vi "thermal_optical_camera_2.vi"() -> ()   [LabVIEW 2025]
panel:
  out "file name out":string
  in  "File Path":string="C:\\Digambar\\Metal_thin_wall\\Optical_images\\Optical_images"
  in  "Stop (F)":bool
  in  "Acquisition Control:\nExposure Time [100, 3E7]":dbl=999.0 caption="Acquisition Control::Exposure Time" min=100.0 max=29999995.0
  in  "Analog Control:\nGain [0, 27]":dbl caption="Analog Control::Gain" min=0.0 max=27.045663671679687
  in  "Analog Control:\nBlack Level [-5, 10]":dbl caption="Analog Control::Black Level" min=-5.0000011920928955 max=10.000002384185791
  in  "Analog Control:\nGamma [0.25, 4.00]":dbl=0.800048828125 caption="Analog Control::Gamma" min=0.25 max=4.0 step=0.05
  out "Optical camera":T1(plugin-control)
  in  "optical capture interval (s)":dbl
  in  "thermal capture interval (s)":dbl
  out "Thermal camera":T1(plugin-control)
  out "IP address":string
  out "Output":string
  in  "Flag Button":bool
  in  "Stop Recording":bool
  in  "Stop Preview":bool
  in  "Focus":dbl(slide) scale=0.0..100.0
  in  "Record":bool
  # "Destination for Optical Images:"
  # "change folder names each time you run,\nso it saves data sets in dedicated folders:\nfolder1\nfolder2\nfolder3\netc..."
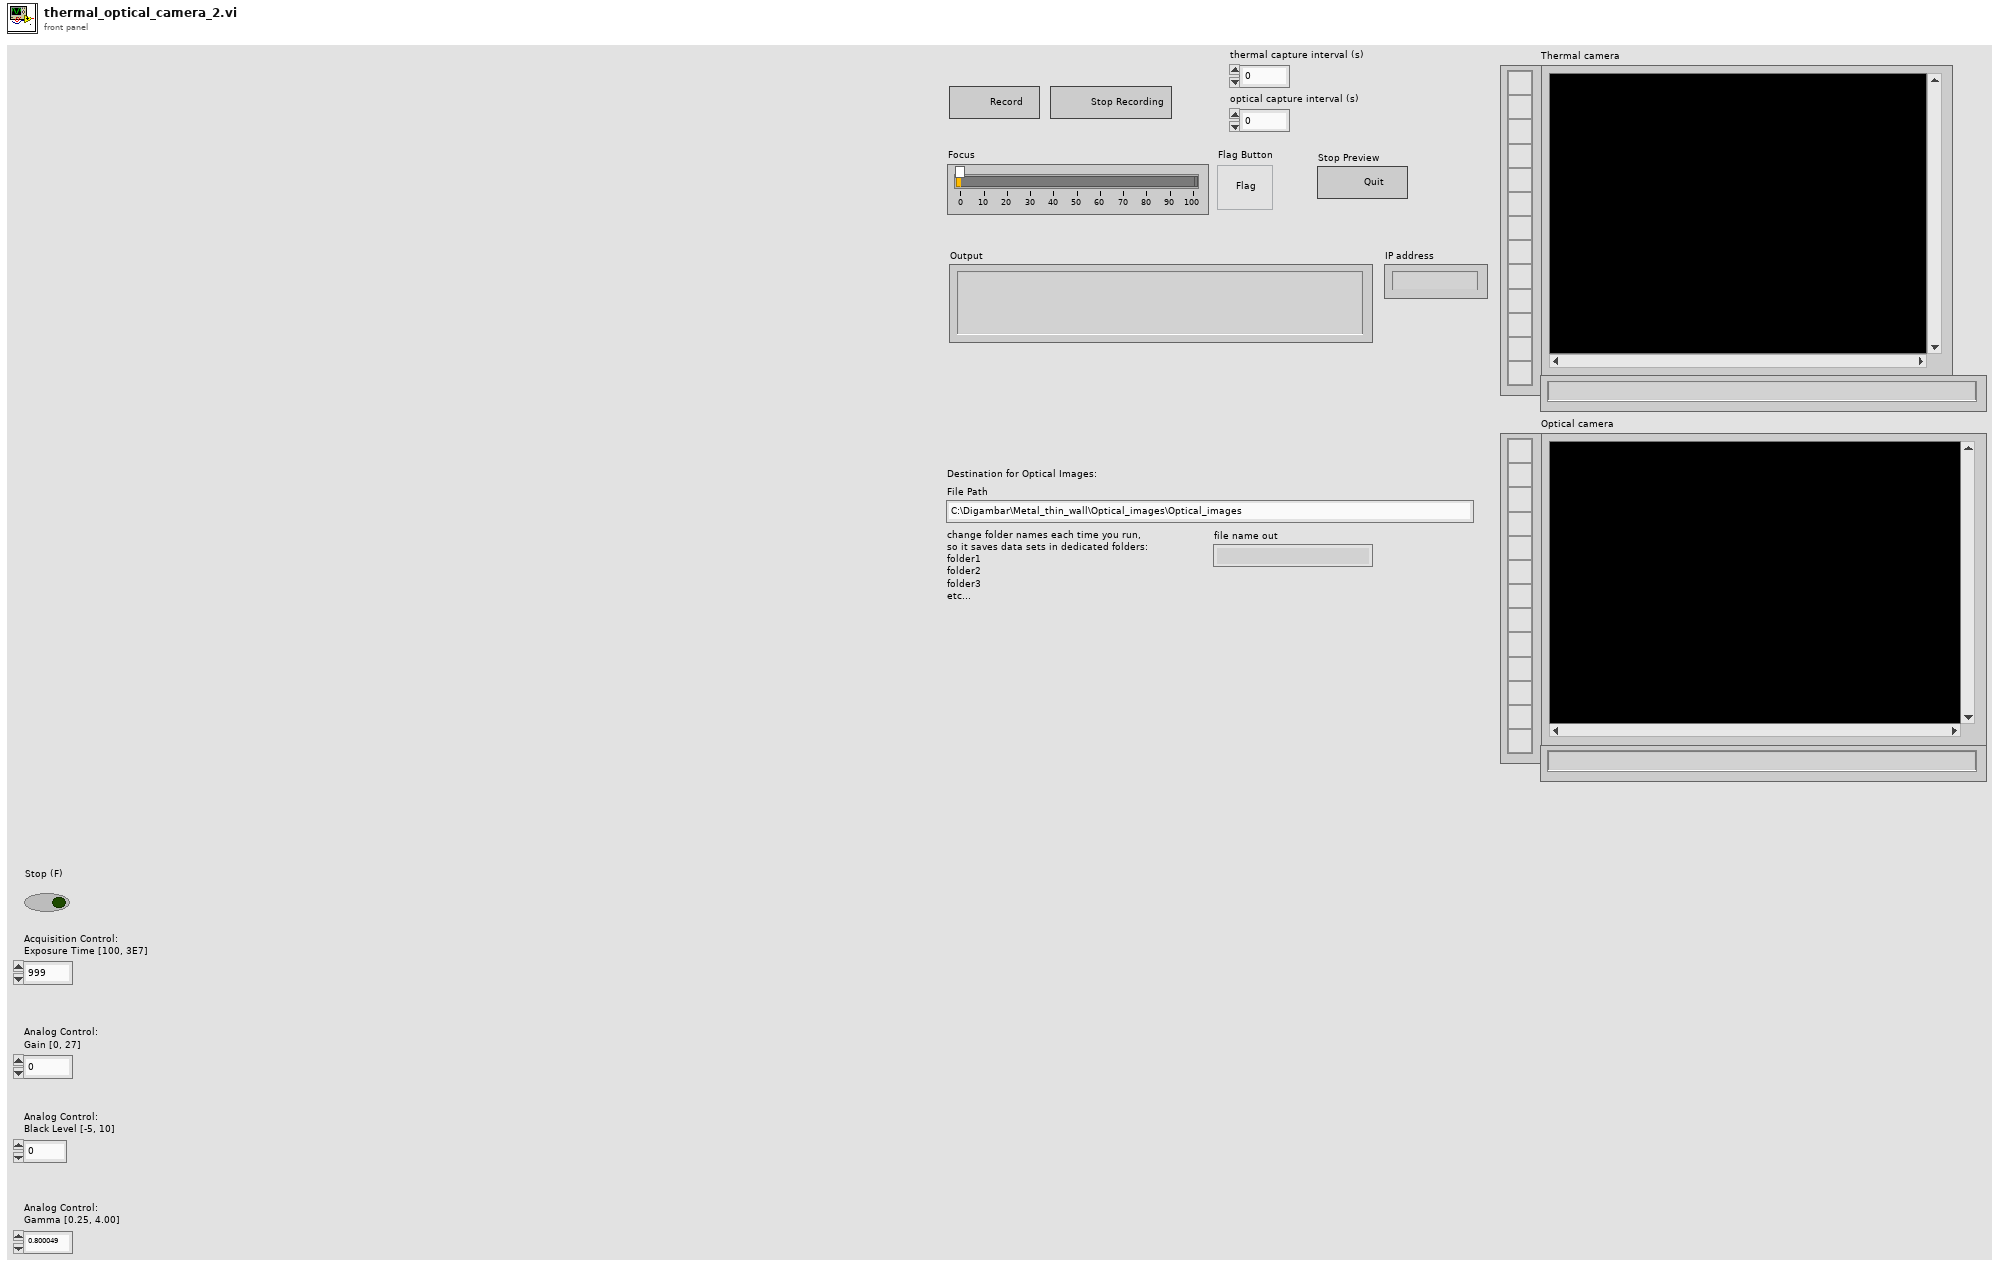
[diagram p1: front panel]
types:
  T1 = typedef "IMAQ Image.ctl" = refnum<image>
  T2 = enum16{"open", "replace", "create", "open or create", "replace or create", "replace or create with confirmation"}
  T3 = enum16{"big-endian, network order", "native, host order", "little-endian"}
  T4 = enum16{"Standard", "Buffered", "CRLF", "Immediate"}
  T5 = typedef "Image Type" = u32
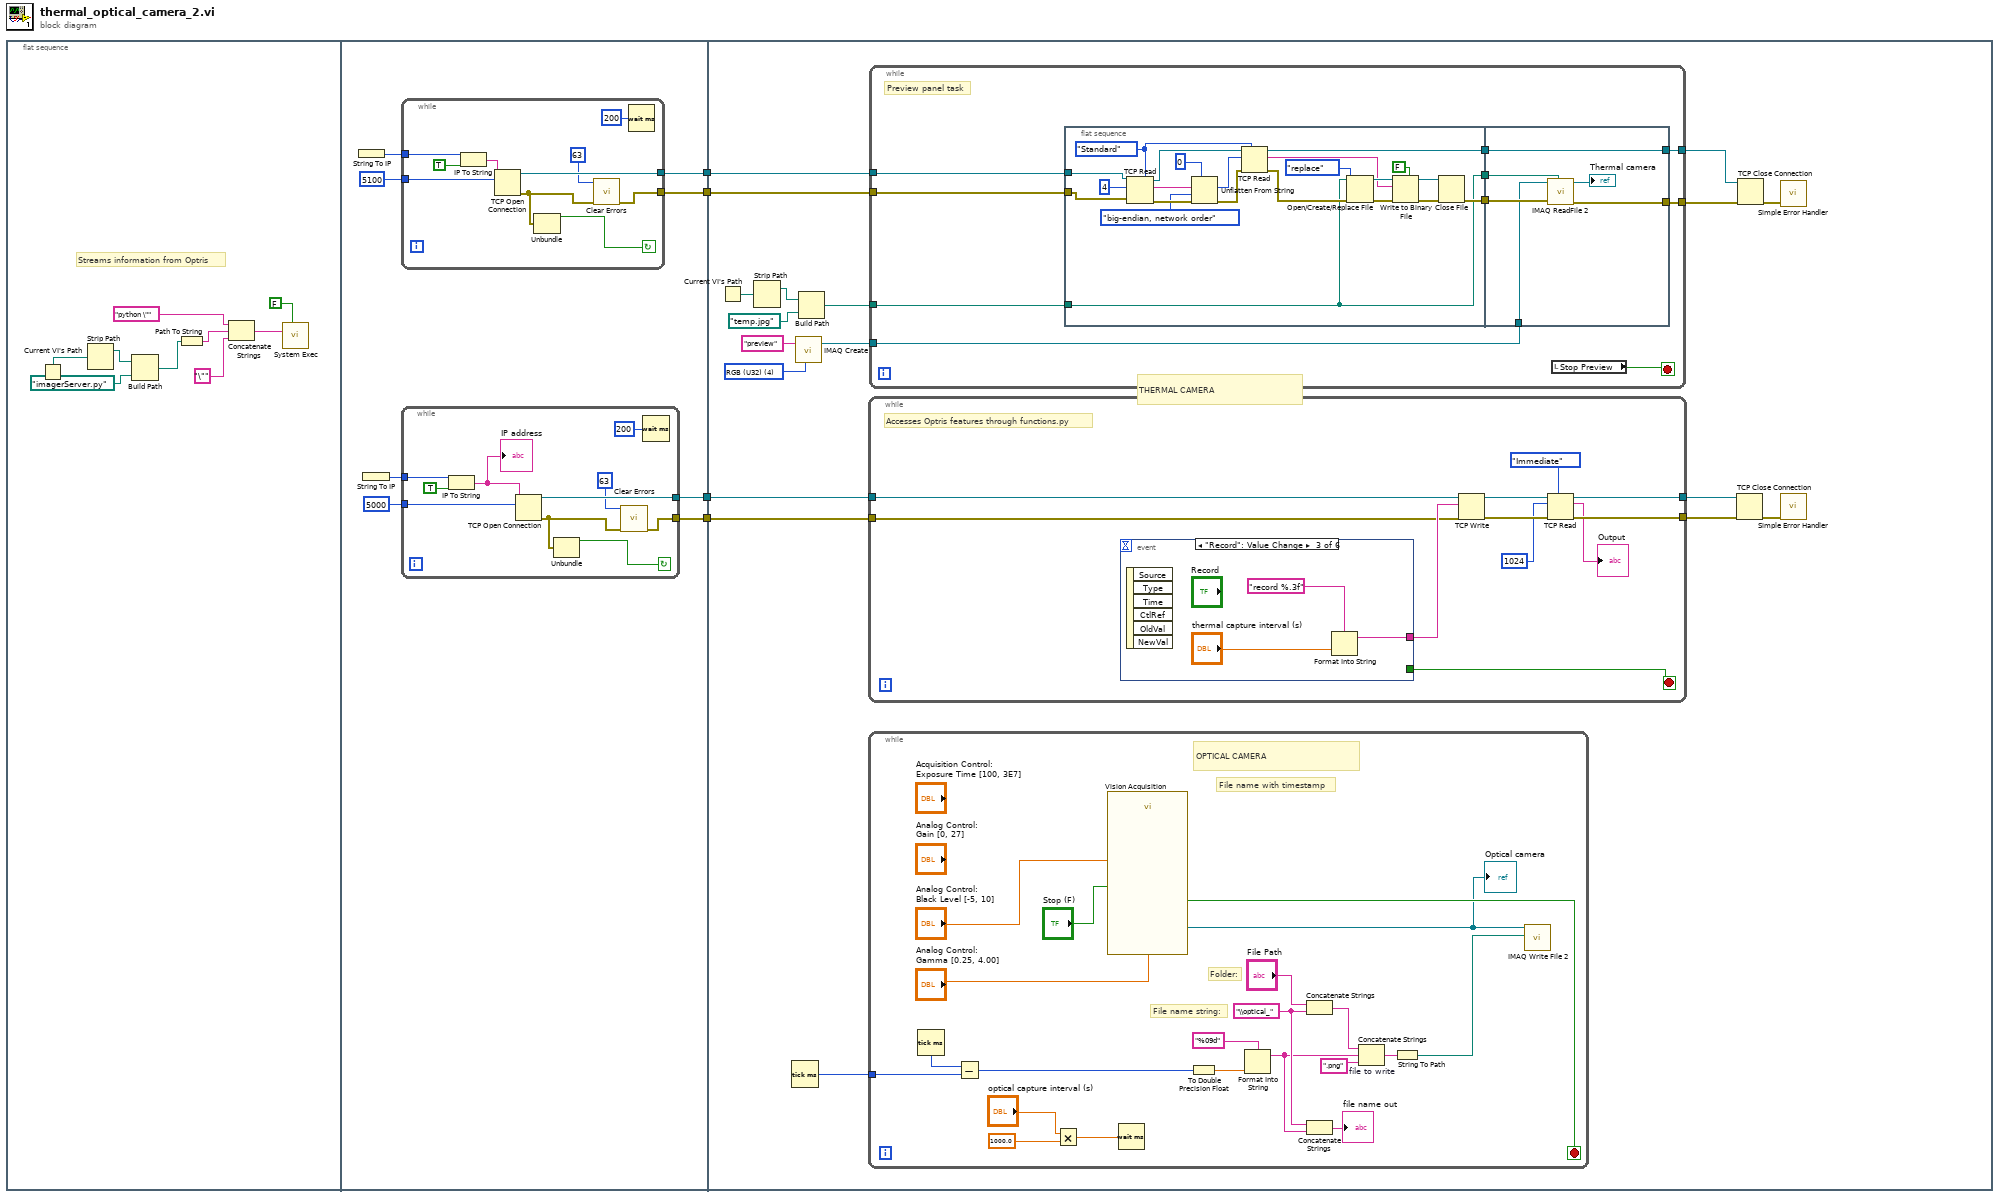
[diagram p0: block diagram]
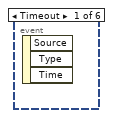
[diagram p2: hidden frame]
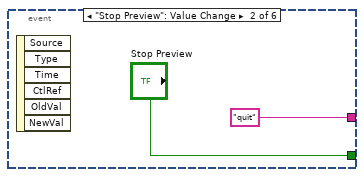
[diagram p3: hidden frame]
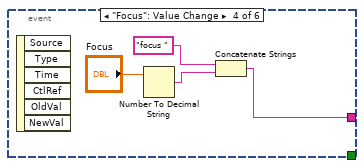
[diagram p4: hidden frame]
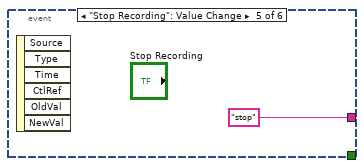
[diagram p5: hidden frame]
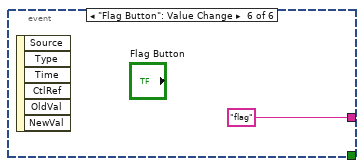
[diagram p6: hidden frame]
diagram:
  n1 = flat-sequence {
    tunnel: [w19] -> w4
    tunnel: [w18] -> w3
    tunnel: [w15] -> w2
    tunnel: [w14] -> w1
    tunnel: w4 -> [w45]
    tunnel: w3 -> [w44]
    tunnel: w2 -> [w43]
    tunnel: w1 -> [w42]
    frame #0 {
      # "Streams information from Optris"
      n2 = Current VI's Path() -> (path=w8:path)
      n3 = Strip Path(path=w8) -> (stripped path=w9:path)  [unwired: 1 out]
      n4 = Build Path(base path=w9, name or relative path=path "imagerServer.py") -> (appended path=w6:path)
      n5 = Path To String(path=w6) -> (string=w12:string)
      n6 = Concatenate Strings("python \"" ("string"), w12, "\"" ("string")) -> (w11:string)
      n7 = call <vilib>:"System Exec.vi"("wait until completion? (T)"=FALSE, "command line"=w11) -> ()  [unwired: 6 in, 4 out]
    }
    frame #1 {
      n8 = String To IP() -> (0:w21:u32)  [unwired: 1 in]
      n9 = String To IP() -> (0:w17:u32)  [unwired: 1 in]
      n10 = while {
        tunnel: [w25] -> w15
        tunnel: [w31] -> w14
        tunnel: w17 -> [w29]
        tunnel: u16 5000 ("remote port or service name") -> [w27]
        stop <- w22 continue-if-true
        n11 = IP To String(1:TRUE ("dot notation? (F)"), 2:w29) -> (0:w30:string)
        "IP address" <- w30
        n12 = TCP Open Connection(address=w30, remote port or service name=w27) -> (connection ID=w31:refnum<k5>, error out=w26:errorcluster)  [unwired: 3 in]
        n13 = Unbundle(w26) -> ("status"=w22:bool)  [unwired: 2 out]
        n14 = call <vilib>:"Clear Errors.vi"("error in (no error)"=w26, "specific error code to clear (0: all)"=63) -> ("error out"=w25:errorcluster)  [unwired: 4 in, 1 out]
        n15 = Wait (ms)(milliseconds to wait=u32 200) -> ()  [unwired: 1 out]
      }
      n16 = while {
        tunnel: w21 -> [w41]
        tunnel: [w35] -> w19
        tunnel: [w39] -> w18
        tunnel: u16 5100 ("remote port or service name") -> [w37]
        stop <- w32 continue-if-true
        n17 = IP To String(1:TRUE ("dot notation? (F)"), 2:w41) -> (0:w40:string)
        n18 = TCP Open Connection(address=w40, remote port or service name=w37) -> (connection ID=w39:refnum<k5>, error out=w36:errorcluster)  [unwired: 3 in]
        n19 = Unbundle(w36) -> ("status"=w32:bool)  [unwired: 2 out]
        n20 = call <vilib>:"Clear Errors.vi"("error in (no error)"=w36, "specific error code to clear (0: all)"=63) -> ("error out"=w35:errorcluster)  [unwired: 4 in, 1 out]
        n21 = Wait (ms)(milliseconds to wait=u32 200) -> ()  [unwired: 1 out]
      }
    }
    frame #2 {
      w47 = T5 4 items=["Grayscale (U8)", "Grayscale (I16)", "Grayscale (SGL)", "Complex (CSG)", "RGB (U32)", "HSL (U32)", "RGB (U64)", "Grayscale (U16)"] ("Image Type")
      # "THERMAL CAMERA"
      n22 = Current VI's Path() -> (path=w58:path)
      n23 = Strip Path(path=w58) -> (stripped path=w59:path)  [unwired: 1 out]
      n24 = Tick Count (ms)() -> (millisecond timer value=w46:u32)
      n25 = call "IMAQ Create"("Image Name"="preview", "Image Type"=w47) -> ("New Image"=w54:T1)  [unwired: 3 in, 1 out]
      n26 = Build Path(base path=w59, name or relative path=path "temp.jpg") -> (appended path=w57:path)
      n27 = while {
        tunnel: [w128] -> w50
        tunnel: [w126] -> w51
        tunnel: w43 -> [w120]
        tunnel: w42 -> [w119]
        stop <- w121 stop-if-true
        # "Accesses Optris features through functions.py"
        n28 = event shown="[2] \"Record\": Value Change" {
          selector: _ -> [_ _ _ _ _ _]
          dyn-events: _ -> [_ _ _ _ _ _]
          timeout: _ -> [_ _ _ _ _ _]
          tunnel: [_ "quit" w134 w136 "stop" "flag"] -> w125
          tunnel: [_ "Stop Preview" _ _ _ _] -> w121
          event Timeout {
            n29 = event-data() -> ()  [unwired: 1 in, 3 out]
          }
          event "Stop Preview": Value Change {
            n30 = event-data() -> ()  [unwired: 1 in, 6 out]
          }
          event "Record": Value Change {
            n31 = event-data() -> ()  [unwired: 1 in, 6 out]
            n32 = Format Into String(format string="record %.3f", "thermal capture interval (s)") -> (resulting string=w134:string)  [unwired: 2 in, 1 out]
          }
          event "Focus": Value Change {
            n33 = event-data() -> ()  [unwired: 1 in, 6 out]
            n34 = Number To Decimal String(number="Focus") -> (decimal integer string=w138:string)  [unwired: 1 in]
            n35 = Concatenate Strings("focus ", w138) -> (w136:string)
          }
          event "Stop Recording": Value Change {
            n36 = event-data() -> ()  [unwired: 1 in, 6 out]
          }
          event "Flag Button": Value Change {
            n37 = event-data() -> ()  [unwired: 1 in, 6 out]
          }
        }
        n38 = TCP Write(connection ID=w119, data in=w125, error in (no error)=w120) -> (connection ID out=w127:refnum<k5>, error out=w129:errorcluster)  [unwired: 1 in, 1 out]
        n39 = TCP Read(connection ID=w127, bytes to read=1024, error in (no error)=w129, 7:T4."Immediate" ("mode (standard)")) -> (connection ID out=w126:refnum<k5>, data out=→"Output":string, error out=w128:errorcluster)  [unwired: 1 in]
      }
      n40 = while {
        tunnel: w46 -> [w68]
        stop <- w79 stop-if-true
        w65 = "\\optical_" ("string")
        # "OPTICAL CAMERA"
        # "File name with timestamp"
        # "Folder:"
        # "File name string:"
        n41 = Tick Count (ms)() -> (millisecond timer value=w69:u32)
        n42 = Subtract(x=w69, y=w68) -> (x-y=w60:u32)
        n43 = Multiply(x="optical capture interval (s)", y=1000.0) -> (x*y=w73:dbl)
        n44 = call "Vision Acquisition"("Analog Control::Black Level"="Analog Control:\nBlack Level [-5, 10]", "Analog Control::Gamma"="Analog Control:\nGamma [0.25, 4.00]", "Stop (F)"="Stop (F)") -> ("Image Out"=w78:T1, "Stopped"=w79:bool)  [unwired: 22 in, 1 out]
        "Optical camera" <- w78
        n45 = Wait (ms)(milliseconds to wait=w73) -> ()  [unwired: 1 out]
        n46 = To Double Precision Float(number=w60) -> (double precision float=w61:dbl)
        n47 = Format Into String(format string="%09d" ("time format string (%c)"), w61) -> (resulting string=w63:string)  [unwired: 2 in, 1 out]
        n48 = Concatenate Strings("File Path", w65) -> (w66:string)
        n49 = Concatenate Strings(w65, w63) -> (→"file name out":string)
        n50 = Concatenate Strings "file to write"(w66, w63, ".png" ("string")) -> (w75:string)
        n51 = String To Path(string=w75) -> (path=w71:path)
        n52 = call-poly "IMAQ Write File 2"("File Path"=w71, "Image"=w78) -> ()  [unwired: 8 in, 2 out]
      }
      n53 = while {
        tunnel: w54 -> [w85]
        tunnel: [w86] -> w55
        tunnel: [w90] -> w56
        tunnel: w57 -> [w88]
        tunnel: w45 -> [w82]
        tunnel: w44 -> [w81]
        stop <- w83 stop-if-true
        # "Preview panel task"
        n54 = flat-sequence {
          tunnel: w88 -> [w94]
          tunnel: [w96] -> w89
          tunnel: [w95] -> w87
          tunnel: [w94] -> w84
          tunnel: w82 -> [w92]
          tunnel: w81 -> [w91]
          tunnel: [w118] -> w90
          tunnel: w89 -> [w118]
          tunnel: w87 -> [w117]
          tunnel: [w116] -> w86
          tunnel: w85 -> [w115]
          tunnel: w84 -> [w114]
          frame #0 {
            w105 = T4."Standard" ("mode (standard)")
            n55 = TCP Read(connection ID=w91, bytes to read=4, error in (no error)=w92, 7:w105) -> (connection ID out=w108:refnum<k5>, data out=w93:string, error out=w111:errorcluster)  [unwired: 1 in]
            n56 = Unflatten From String(type=0, binary string=w93, byte order (0:big-endian, network order)=T3."big-endian, network order", error in (no error)=w111) -> (value=w106:i32, error out=w107:errorcluster)  [unwired: 1 in, 1 out]
            n57 = TCP Read(connection ID=w108, bytes to read=w106, error in (no error)=w107, 7:w105) -> (connection ID out=w96:refnum<k5>, data out=w101:string, error out=w103:errorcluster)  [unwired: 1 in]
            n58 = Open/Create/Replace File(file path (use dialog)=w94, error in=w103, operation (0:open)=T2."replace") -> (refnum out=w102:refnum<file>, error out=w99:errorcluster)  [unwired: 3 in, 1 out]
            n59 = Write to Binary File(file (use dialog)=w102, data=w101, error in=w99, 5:FALSE ("prepend array or string size? (T)")) -> (refnum out=w97:refnum<file>, error out=w98:errorcluster)  [unwired: 2 in, 1 out]
            n60 = Close File(refnum=w97, error in=w98) -> (error out=w95:errorcluster)  [unwired: 1 out]
          }
          frame #1 {
            n61 = call "IMAQ ReadFile 2"("File Path"=w114, "error in (no error)"=w117, "Image"=w115) -> ("error out"=w116:errorcluster, "Image Out"=→"Thermal camera":T1)  [unwired: 4 in, 3 out]
          }
        }
        n62 = local read "Stop Preview"() -> (w83:bool)
      }
      n63 = TCP Close Connection(connection ID=w51, error in (no error)=w50) -> (error out=w52:errorcluster)  [unwired: 1 in, 1 out]
      n64 = TCP Close Connection(connection ID=w56, error in (no error)=w55) -> (error out=w53:errorcluster)  [unwired: 1 in, 1 out]
      n65 = call <vilib>:"Simple Error Handler.vi"("error in (no error)"=w53) -> ()  [unwired: 4 in, 5 out]
      n66 = call <vilib>:"Simple Error Handler.vi"("error in (no error)"=w52) -> ()  [unwired: 4 in, 5 out]
    }
  }
